vi "_Set Cell DataType.vi"(8 "error in":errorcluster, 10 "Datatype":i32(ring) items=["Boolean", "Number", "Error", "SharedString", "String", "InlineString", "Date"], 11 "Cell in":refnum<k24>) -> (0 "error out":errorcluster, 3 "Cell out":refnum<k24>)   [LabVIEW 2021, in "Open Xml.lvlib"]
uses:
  Open Xml.lvlib
  D:/git/Open-Xml-LabVIEW/dll/DocumentFormat.OpenXml.dll
  dll/DocumentFormat.OpenXml.dll
  D:/git/Open-Xml-LabVIEW/dll/OpenXmlGenericsWrapper.dll
  dll/OpenXmlGenericsWrapper.dll
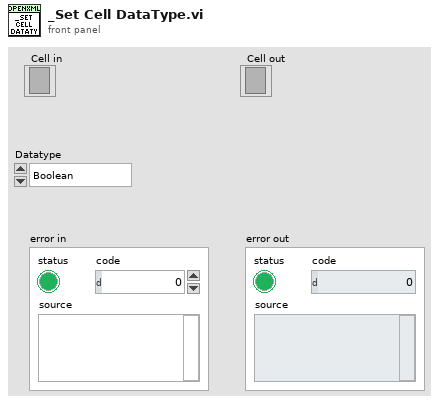
[diagram p1: front panel]
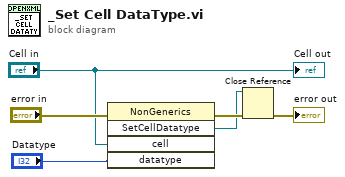
[diagram p0: block diagram]
diagram:
  n1 = invoke class="NonGenerics" method="SetCellDatatype"(error in="error in", "cell"="Cell in", "datatype"="Datatype") -> (error out=w6:errorcluster, "SetCellDatatype"=w2:refnum<k24>)  [unwired: 2 in, 3 out]
  n2 = Close Reference(reference=w2, error in (no error)=w6) -> (error out=→"error out":errorcluster)
  "Cell out" <- "Cell in"
